vi "Origin_or_TempCoordinate.vi"(0 "Origin":T1, 2 "Temp Coord":T1) -> (10 "Temp?":bool, 21 "Origin out":T1)   [LabVIEW 2020]
uses:
  <vilib>/Utility/miscctls.llb/LVPoint32TypeDef.ctl
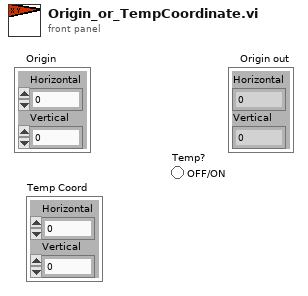
[diagram p1: front panel]
types:
  T1 = typedef "LVPoint32TypeDef.ctl" = cluster{"Horizontal":i32, "Vertical":i32}
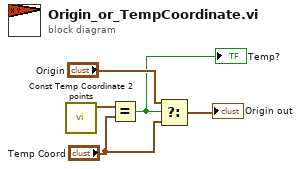
[diagram p0: block diagram]
diagram:
  n1 = call "Const Temp Coordinate 2 points.vi"() -> ("Const Temp Coordinate"=w5:T1)  [unwired: 11 out]
  n2 = Equal?(x=w5, y="Temp Coord") -> (x = y?=w1:bool)
  "Temp?" <- w1
  n3 = Select(t="Origin", s=w1, f="Temp Coord") -> (s? t:f=→"Origin out":T1)
